vi "Final_Log.vi"() -> ()   [LabVIEW 2016]
panel:
  out "Natural Log":ext
  out "log2X":ext
  in  "X":dbl
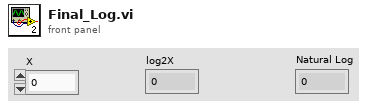
[diagram p1: front panel]
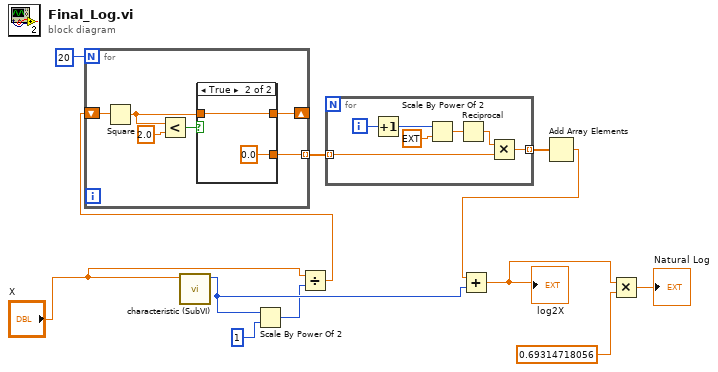
[diagram p0: block diagram]
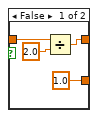
[diagram p2: hidden frame]
diagram:
  n1 = call "characteristic (SubVI).vi"("Input"="X") -> ("Numeric"=w7:i32)  [unwired: 10 in]
  n2 = Scale By Power Of 2(n=w7, x=1 ("n")) -> (x*2^n=w5:i32)
  n3 = Divide(x="X", y=w5) -> (x/y=w6:dbl)
  n4 = for {
    N: 20 ("Numeric 2") -> [_]
    shift-right: [w15] -> _
    shift-left: w6 -> [w18]
    tunnel: [w13] -> w11 mode=indexing
    n5 = Square(x=w18) -> (x^2=w14:dbl)
    n6 = Less?(x=w14, y=2.0) -> (x < y?=w16:bool)
    n7 = case shown="True" w16 {
      tunnel: [w20 w24] -> w15
      tunnel: w14 -> [w22 w24]
      tunnel: [1.0 ("Numeric") 0.0 ("Numeric")] -> w13
      frame False {
        n8 = Divide(x=w22, y=2.0) -> (x/y=w20:dbl)
      }
      frame True {
      }
    }
  }
  n9 = for {
    tunnel: w11 -> [w25] mode=indexing
    tunnel: [w26] -> w10 mode=indexing
    i -> [w29]
    n10 = Increment(x=w29) -> (x+1=w28:i32)
    n11 = Scale By Power Of 2(n=w28, x=ext 1.0) -> (x*2^n=w31:ext)
    n12 = Reciprocal(x=w31) -> (1/x=w27:ext)
    n13 = Multiply(x=w27, y=w25) -> (x*y=w26:ext)
  }
  n14 = Add Array Elements(numeric array=w10) -> (sum=w8:ext)
  n15 = Add(x=w8, y=w7) -> (x+y=w4:ext)
  "log2X" <- w4
  n16 = Multiply(x=w4, y=0.69314718056 ("Numeric")) -> (x*y=→"Natural Log":ext)
